vi "Configure Clock 5772_v1.vi"(8 "error in":errorcluster, 10 "Clock Source":T2(ring), 11 "FPGA VI Reference In":T1) -> (0 "error out":errorcluster, 2 "Configuration Error":bool, 3 "FPGA VI Reference Out":T1)   [LabVIEW 2015, in "7976R_v1.lvclass"]
doc: "This VI configures the clock source for the NI 5772. For execution steps, refer to the comments on the block diagram."
uses:
  <userlib>/SE-APP-Receiver/NI5772/7976R_v1/7976R_v1.lvclass
  <userlib>/SE-APP-Receiver/NI5772/7976R_v1/Private/FPGA VI Reference_DDC_v1.8.ctl
  <vilib>/Utility/error.llb/Error Cluster From Error Code.vi
  <vilib>/rvi/errors/niLvFpgaAdjustHostInterfaceError.vi
  <vilib>/rvi/interface/nirviReadWriteControl/nirviReadWriteControl.xnode
  <vilib>/rvi/interface/Simulation/niFpgaSimulationCallBeginRW.vi
  NiFpgaLv.dll
panel:
  # "This VI configures the clock source for the NI 5771. For execution steps, refer to the comments on the block diagram."
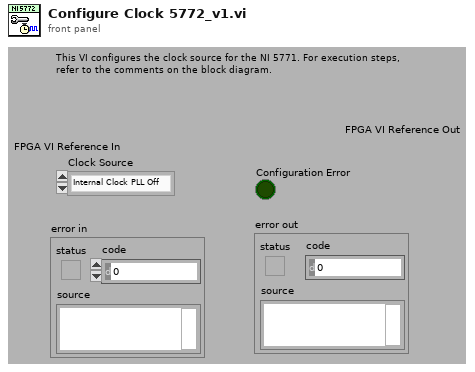
[diagram p1: front panel]
types:
  T1 = typedef "7976R_v1.lvclass/FPGA VI Reference_DDC_v1.8.ctl" = refnum<k20>
  T2 = enum8{"Internal Clock PLL Off", "Internal Clock PLL On (REF IN)", "External Clock (CLK_IN)", "Internal Clock PLL On (IoModSyncClk)"}
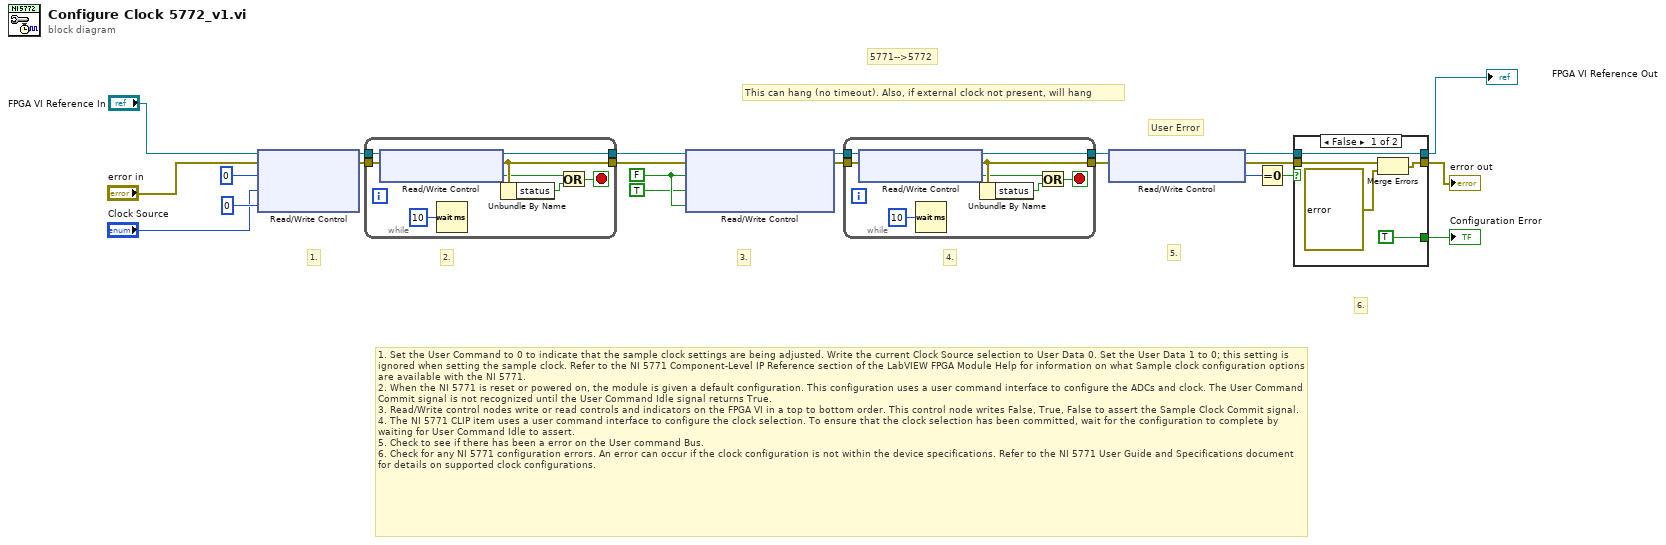
[diagram p0: block diagram]
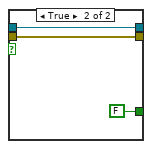
[diagram p2: hidden frame]
diagram:
  w17 = FALSE ("Sample Clock Commit")
  # "User Error"
  # "5771-->5772"
  # "This can hang (no timeout). Also, if external clock not present, will hang"
  # "6."
  # "1. Set the User Command to 0 to indicate that the sample clock settings are being adjusted. Write the current Clock Source selection to User Data 0. Set the User Data 1 to 0; this setting is ignored when setting the sample clock. Refer to the NI 5771 Component-Level IP Reference section of the LabVIEW FPGA Module Help for information on what Sample clock configuration options are available with the NI 5771.\n2. When the NI 5771 is reset or powered on, the module is given a default configuration. This configuration uses a user command interface to configure the ADCs and clock. The User Command Commit signal is not recognized until the User Command Idle signal returns True.\n3. Read/Write control nodes write or read controls and indicators on the FPGA VI in a top to bottom order. This control node writes False, True, False to assert the Sample Clock Commit signal.\n4. The NI 5771 CLIP item uses a user command interface to configure the clock selection. To ensure that the clock selection has been committed, wait for the configuration to complete by waiting for User Command Idle to assert.\n5. Check to see if there has been a error on the User command Bus. \n6. Check for any NI 5771 configuration errors. An error can occur if the clock configuration is not within the device specifications. Refer to the NI 5771 User Guide and Specifications document for details on supported clock configurations."
  # "5."
  # "4."
  # "3."
  # "2."
  # "1."
  n1 = xnode "Read/Write Control"("FPGA VI Reference In"="FPGA VI Reference In", "error in"="error in", "User Command"=u8 0, "User Data 0"="Clock Source", "User Data 1"=u8 0) -> ("FPGA VI Reference Out"=w21:T1, "error out"=w20:errorcluster)
  n2 = while {
    tunnel: w21 -> [w26]
    tunnel: w20 -> [w27]
    tunnel: [w24] -> w18
    tunnel: [w25] -> w19
    stop <- w28 stop-if-true
    n3 = xnode "Read/Write Control"("FPGA VI Reference In"=w26, "error in"=w27) -> ("FPGA VI Reference Out"=w25:T1, "error out"=w24:errorcluster, "User Command Idle"=w23:bool)
    n4 = Wait (ms)(milliseconds to wait=u32 10) -> ()  [unwired: 1 out]
    n5 = Unbundle By Name(w24) -> ("status"=w29:bool)
    n6 = Or(x=w23, y=w29) -> (x .or. y?=w28:bool)
  }
  n7 = xnode "Read/Write Control"("FPGA VI Reference In"=w19, "error in"=w18, "User Command Commit"=w17, "User Command Commit"=TRUE ("Sample Clock Commit"), "User Command Commit"=w17) -> ("FPGA VI Reference Out"=w15:T1, "error out"=w14:errorcluster)
  n8 = while {
    tunnel: w15 -> [w34]
    tunnel: w14 -> [w35]
    tunnel: [w32] -> w13
    tunnel: [w33] -> w12
    stop <- w36 stop-if-true
    n9 = xnode "Read/Write Control"("FPGA VI Reference In"=w34, "error in"=w35) -> ("FPGA VI Reference Out"=w33:T1, "error out"=w32:errorcluster, "User Command Idle"=w31:bool)
    n10 = Wait (ms)(milliseconds to wait=u32 10) -> ()  [unwired: 1 out]
    n11 = Unbundle By Name(w32) -> ("status"=w37:bool)
    n12 = Or(x=w31, y=w37) -> (x .or. y?=w36:bool)
  }
  n13 = xnode "Read/Write Control"("FPGA VI Reference In"=w12, "error in"=w13) -> ("FPGA VI Reference Out"=w5:T1, "error out"=w9:errorcluster, "User Command Status"=w8:u8)
  n14 = Equal To 0?(x=w8) -> (x = 0?=w7:bool)
  n15 = case shown="False" w7 {
    tunnel: [w43 w46] -> w4
    tunnel: w9 -> [w42 w46]
    tunnel: [TRUE ("Configured?") FALSE ("Configured?")] -> w3
    tunnel: w5 -> [w39 w44]
    tunnel: [w39 w44] -> w1
    frame False {
      n16 = Merge Errors(w42, errorcluster {"status"=TRUE, "code"=-8998, "source"="IO Module clock not configured correctly. Please ensure that the desired clock meets the required specifications."} ("error in")) -> (w43:errorcluster)
    }
    frame True {
    }
  }
  "error out" <- w4
  "Configuration Error" <- w3
  "FPGA VI Reference Out" <- w1
